vi "Do Insertion.vi"(8 "error in (no error)":errorcluster, 9 "Insertion Request Time":timestamp, 10 "Viewable":refnum<class "IViewable.lvclass">, 11 "ProtectedSubpanel in":refnum<class "ProtectedSubpanel.lvclass">) -> (0 "error out":errorcluster, 2 "Viewable Out":refnum<class "IViewable.lvclass">, 3 "ProtectedSubpanel out":refnum<class "ProtectedSubpanel.lvclass">)   [LabVIEW 2015, in "IViewable.lvlib" / "ProtectedSubpanel.lvclass"]
uses:
  ProtectedSubpanel.lvclass
  IViewable/IViewable.lvclass
  ProtectedSubpanel.lvclass/ProtectedSubpanel.ctl
  <vilib>/ActorFramework/Actor/Actor.lvclass/Actor.ctl
  <vilib>/ActorFramework/Message Enqueuer/Message Enqueuer.lvclass/Message Enqueuer.ctl
  IViewable/IViewable.lvclass/IViewable.ctl
  <vilib>/ActorFramework/Message Enqueuer/Message Enqueuer.lvclass
  <vilib>/ActorFramework/Actor/Read Self Enqueuer.vi
  <vilib>/ActorFramework/Message Enqueuer/Enqueue.vi
  <vilib>/ActorFramework/Message Enqueuer/Init from Existing Queue.vi
  <vilib>/ActorFramework/Message Priority Queue/Priority Enqueue.vi
  IViewable Messages/Removed From Subpanel Msg/Removed From Subpanel Msg.lvclass
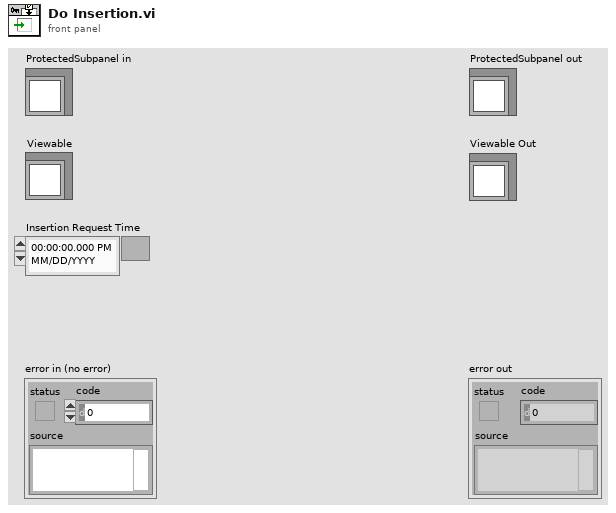
[diagram p1: front panel]
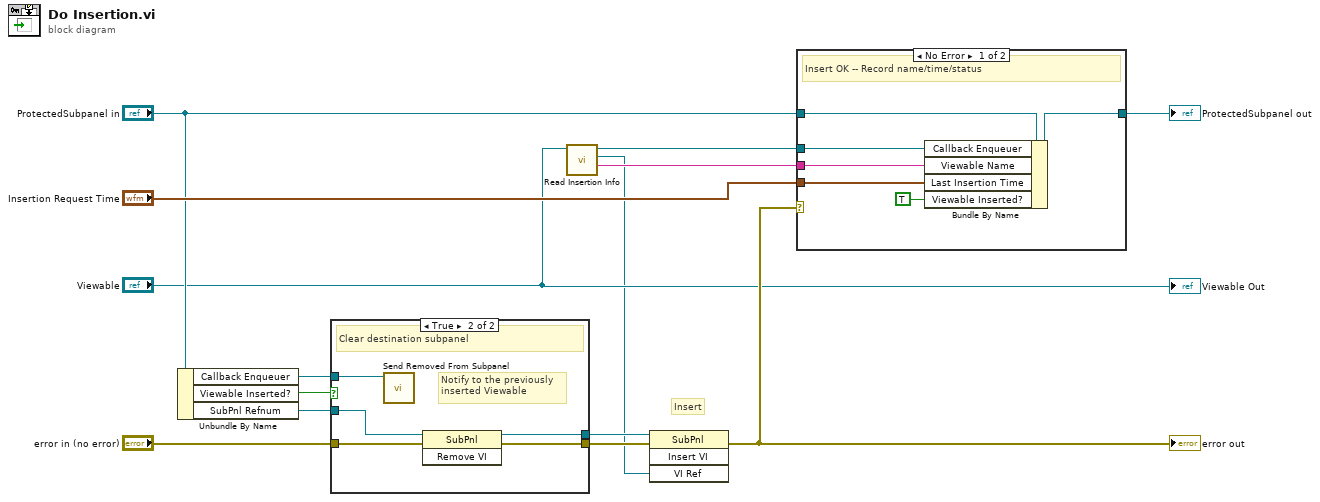
[diagram p0: block diagram]
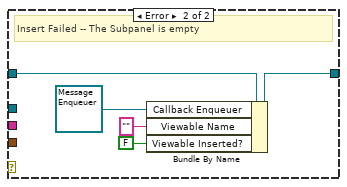
[diagram p3: hidden frame]
diagram:
  # "Insert"
  n1 = Unbundle By Name("ProtectedSubpanel in") -> ("Callback Enqueuer"=w5:refnum<class "Message Enqueuer.lvclass">, "Viewable Inserted?"=w13:bool, "SubPnl Refnum"=w14:refnum<vi>)
  n2 = case shown="True" w13 {
    tunnel: w14 -> [w16 w21]
    tunnel: "error in (no error)" -> [w15 w20]
    tunnel: [w16 w19] -> w12
    tunnel: w5 -> [_ w18]
    tunnel: [w15 w17] -> w2
    frame False {
      # "Subpanel is empty -- Do nothing"
    }
    frame True {
      # "Notify to the previously\ninserted Viewable"
      # "Clear destination subpanel"
      n3 = call "Send Removed From Subpanel.vi"("Message Enqueuer"=w18) -> ()  [unwired: 9 in, 2 out]
      n4 = invoke class="SubPnl" method="Remove VI"(reference=w21, error in=w20) -> (reference out=w19:refnum<vi>, error out=w17:errorcluster)  [unwired: 1 in, 1 out]
    }
  }
  n5 = call "Read Insertion Info.vi"("Viewable in"="Viewable") -> ("Name"=w8:string, "VI Refnum"=w1:refnum<vi>, "Viewable Callback Enqueuer"=w7:refnum<class "Message Enqueuer.lvclass">)  [unwired: 8 in]
  n6 = invoke class="SubPnl" method="Insert VI"(reference=w12, error in=w2, "VI Ref"=w1) -> (error out=w4:errorcluster)  [unwired: 1 in, 3 out]
  "error out" <- w4
  n7 = case shown="No Error" w4 {
    tunnel: [w27 w31] -> w11
    tunnel: "Insertion Request Time" -> [w23 _]
    tunnel: "ProtectedSubpanel in" -> [w26 w32]
    tunnel: w8 -> [w24 _]
    tunnel: w7 -> [w22 _]
    frame No Error {
      # "Insert OK -- Record name/time/status"
      n8 = Bundle By Name(cluster=w26, "Callback Enqueuer"=w22, "Viewable Name"=w24, "Last Insertion Time"=w23, "Viewable Inserted?"=TRUE ("View Inserted?")) -> (w27:refnum<class "ProtectedSubpanel.lvclass">)
    }
    frame Error {
      # "Insert Failed -- The Subpanel is empty"
      n9 = Bundle By Name(cluster=w32, "Callback Enqueuer"=refnum<class "Message Enqueuer.lvclass"> refnum ("Viewable Callback Enqueuer"), "Viewable Name"="" ("Inserted View Name"), "Viewable Inserted?"=FALSE) -> (w31:refnum<class "ProtectedSubpanel.lvclass">)
    }
  }
  "ProtectedSubpanel out" <- w11
  "Viewable Out" <- "Viewable"
